vi "Create Control From Reference.vi"() -> ()   [LabVIEW 2019]
doc: "Demonstrates the Create from Reference method to programmatically create a copy of a control based on its reference."
panel:
  in  "Source Cluster":string="Source Cluster"
  # "Overview: Demonstrates the Create from Reference method to programmatically create a copy of a control based on its reference.\nInstructions:\n1. Open Test - Create from Ref Source.vi and Test - Create from Ref Target.vi.\n2. Run this VI. The Source Cluster on the panel of the source VI will be copied to the panel of the target VI.\n\nNote: The Create from Reference method can be used to copy any control you can obtain a reference to.  This is notable because the New VI Object function can only create a control which has been previously saved to disk."
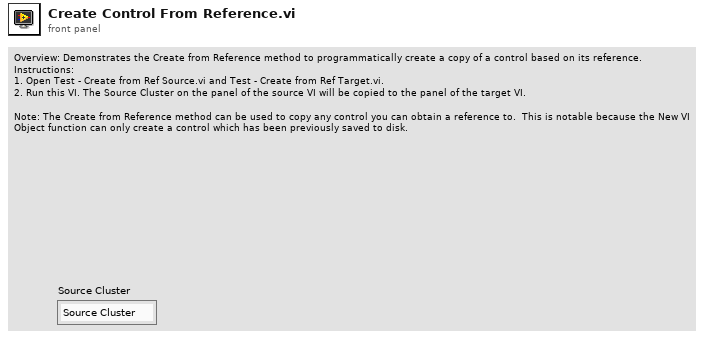
[diagram p1: front panel]
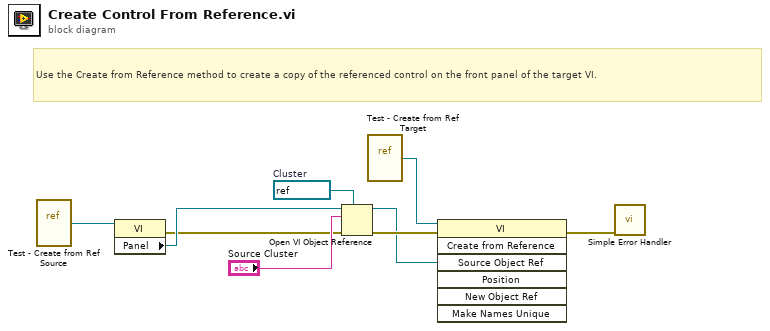
[diagram p0: block diagram]
diagram:
  w5 = refnum<vi> refnum  # Cluster
  # "Use the Create from Reference method to create a copy of the referenced control on the front panel of the target VI."
  n1 = vi-ref "Test - Create from Ref Source.vi"() -> (w8:refnum<vi>)
  n2 = property class="VI"(reference=w8) -> (error out=w4:errorcluster, "Panel"=w7:refnum<vi>)  [unwired: 1 in, 1 out]
  n3 = Open VI Object Reference(7:w5, 8:w4, 10:"Source Cluster", 11:w7) -> (0:w3:errorcluster, 3:w2:refnum<vi>)
  n4 = vi-ref "Test - Create from Ref Target.vi"() -> (w9:refnum<vi>)
  n5 = invoke class="VI" method="Create from Reference"(reference=w9, error in=w3, "Source Object Ref"=w2) -> (error out=w1:errorcluster)  [unwired: 4 in, 6 out]
  n6 = call <vilib>:"Simple Error Handler.vi"("error in (no error)"=w1) -> ()  [unwired: 4 in, 5 out]
